vi "Next_Action_New.vi"(4 "error in (no error)":errorcluster, 6 "Operations":T1, 7 "queue in":refnum<queue>) -> (0 "error out":errorcluster, 1 "No command?":bool, 2 "Operations Out":T1, 3 "queue out":refnum<queue>)   [LabVIEW 2015]
uses:
  ScriptArray.ctl
  Script.ctl
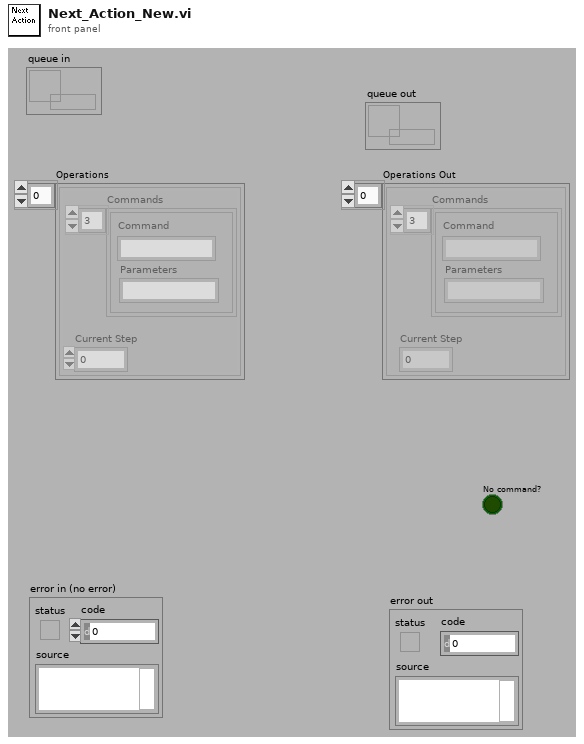
[diagram p1: front panel]
types:
  T1 = typedef "ScriptArray.ctl" = T2[]
  T2 = typedef "Script.ctl" = cluster{"Current Step":i32, "Commands":cluster{"Command":string, "Parameters":string}[]}
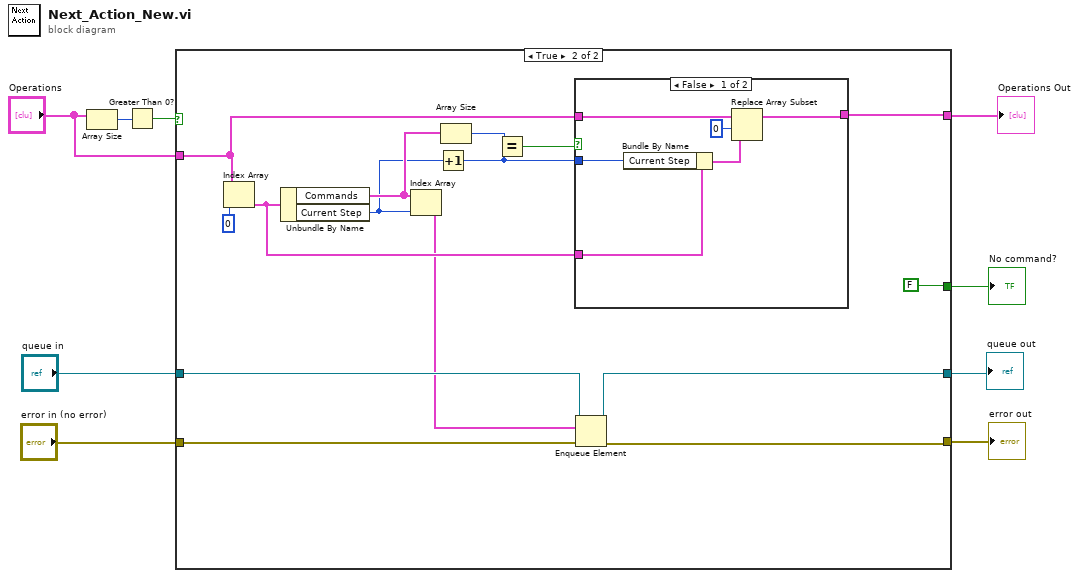
[diagram p0: block diagram]
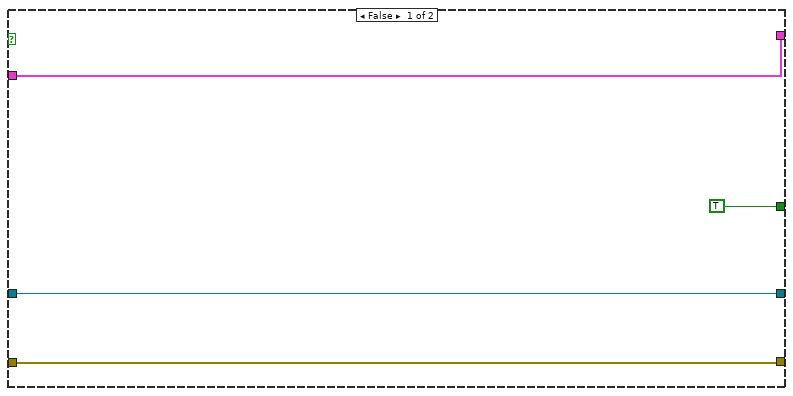
[diagram p2: hidden frame]
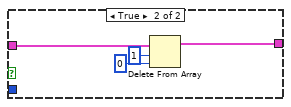
[diagram p3: hidden frame]
diagram:
  n1 = Array Size(array="Operations") -> (size(s)=w9:i32)
  n2 = Greater Than 0?(x=w9) -> (x > 0?=w8:bool)
  n3 = case shown="True" w8 {
    tunnel: "Operations" -> [w13 w24]
    tunnel: "error in (no error)" -> [w12 w21]
    tunnel: [w12 w19] -> w6
    tunnel: [w13 w18] -> w5
    tunnel: "queue in" -> [w11 w20]
    tunnel: [w11 w15] -> w2
    tunnel: [TRUE FALSE] -> w1
    frame False {
    }
    frame True {
      n4 = Index Array(array=w24, index=0) -> (element=w17:T2)
      n5 = Unbundle By Name(w17) -> ("Commands"=w27:cluster{"Command":string, "Parameters":string}[], "Current Step"=w26:i32)
      n6 = Index Array(array=w27, index=w26) -> (element=w16:cluster{"Command":string, "Parameters":string})
      n7 = Increment(x=w26) -> (x+1=w23:i32)
      n8 = Array Size(array=w27) -> (size(s)=w25:i32)
      n9 = Equal?(x=w25, y=w23) -> (x = y?=w22:bool)
      n10 = case shown="False" w22 {
        tunnel: w24 -> [w34 w38]
        tunnel: w23 -> [w29 _]
        tunnel: [w33 w35] -> w18
        tunnel: w17 -> [w30 _]
        frame False {
          n11 = Bundle By Name(cluster=w30, "Current Step"=w29) -> (w31:T2)
          n12 = Replace Array Subset(array=w34, new element=w31, index=0) -> (w33:T1)
        }
        frame True {
          n13 = Delete From Array(array=w38, length=1, index=0) -> (array with subset deleted=w35:T1)  [unwired: 1 out]
        }
      }
      n14 = Enqueue Element(queue=w20, element=w16, error in (no error)=w21) -> (queue out=w15:refnum<queue>, error out=w19:errorcluster)  [unwired: 1 in, 1 out]
    }
  }
  "error out" <- w6
  "Operations Out" <- w5
  "queue out" <- w2
  "No command?" <- w1
